vi "add control module.vi"(6 "output range":cluster{"output high":dbl, "output low":dbl}={"output high"=100.0, "output low"=-100.0}, 8 "error in":errorcluster, 9 "gains":T2, 10 "name":string, 11 "user module configuration in":refnum<class "TEST CONFIGURATION.lvclass">) -> (0 "error out":errorcluster, 1 "generated control module":T1={"name"="", "setpoint"=refnum, "process variable"=refnum, "output"=refnum, "gains"={"Kp"=0.0, "Ki"=0.0, "Kd"=0.0}, "output range"={"output high"=100.0, "output low"=-100.0}} {"output range"."output low" format="%.2f"; "output range"."output high" format="%.2f"}, 2 "generated channels":refnum<class "TBM channel.lvclass">[](array[class]), 3 "user module configuration out":refnum<class "TEST CONFIGURATION.lvclass">)   [LabVIEW 2013, in "configuration tests.lvlib" / "TEST CONFIGURATION.lvclass"]
uses:
  TEST CONFIGURATION.lvclass
  <vilib>/NI/Tag Bus Module Framework/channel/TBM channel.lvclass
  gains.ctl
  control module configuration.ctl
  TEST CONFIGURATION.lvclass/TEST CONFIGURATION.ctl
  <vilib>/NI/Tag Bus Module Framework/channel/channel classification.ctl
  <vilib>/NI/Tag Bus/tag/Data Type.ctl
  <vilib>/NI/Tag Bus/tag/tag descriptor.lvclass
  <vilib>/NI/Configuration Framework/NISE_CEF_TreeControl.lvlib
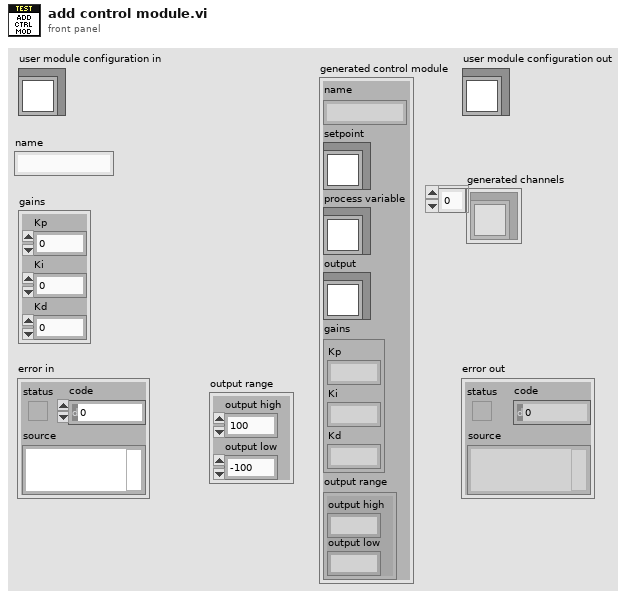
[diagram p1: front panel]
types:
  T1 = typedef "configuration tests.lvlib/TEST CONFIGURATION.lvclass/control module configuration.ctl" = cluster{"name":string, "setpoint":refnum<class "TBM channel.lvclass">, "process variable":refnum<class "TBM channel.lvclass">, "output":refnum<class "TBM channel.lvclass">, "gains":T2, "output range":cluster{"output high":dbl, "output low":dbl}}
  T2 = typedef "configuration tests.lvlib/TEST CONFIGURATION.lvclass/gains.ctl" = cluster{"Kp":dbl, "Ki":dbl, "Kd":dbl}
  T3 = typedef "TBM channel.lvclass/channel classification.ctl" = enum16{"input data", "output data", "processing parameter", "processing result"}
  T4 = typedef "tag bus.lvlib/tag descriptor.lvclass/Data Type.ctl" = enum16{"Double", "Single", "I64", "I32", "I16", "I8", "U64", "U32", "U16", "U8", "Boolean", "String", "Array of Double", "Array of Single", "Array of I64", "Array of I32", "Array of I16", "Array of I8", "Array of U64", "Array of U32", "Array of U16", "Array of U8", "Array of Boolean", "Array of String"}
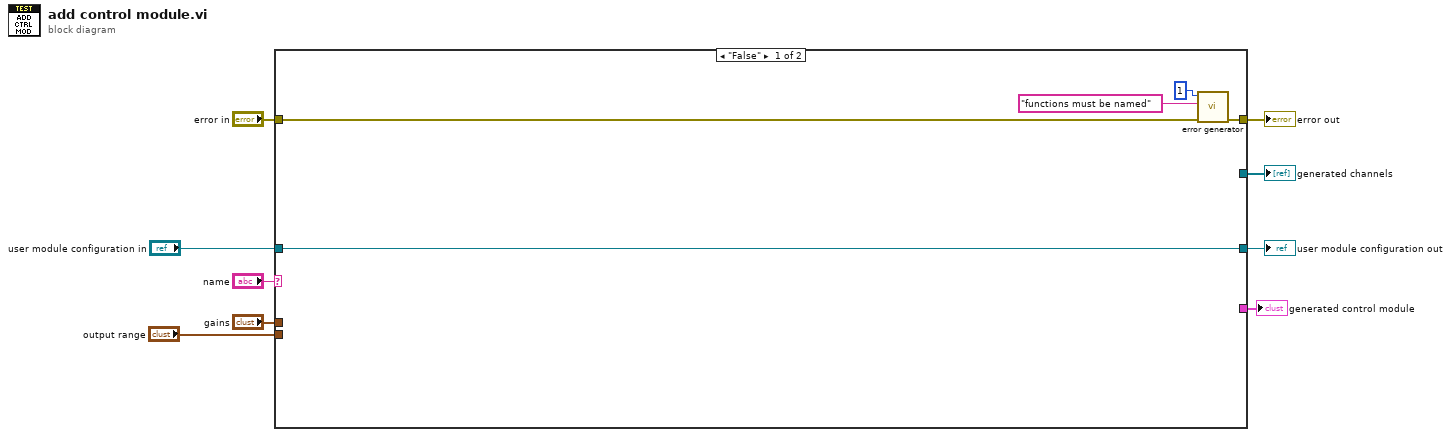
[diagram p0: block diagram]
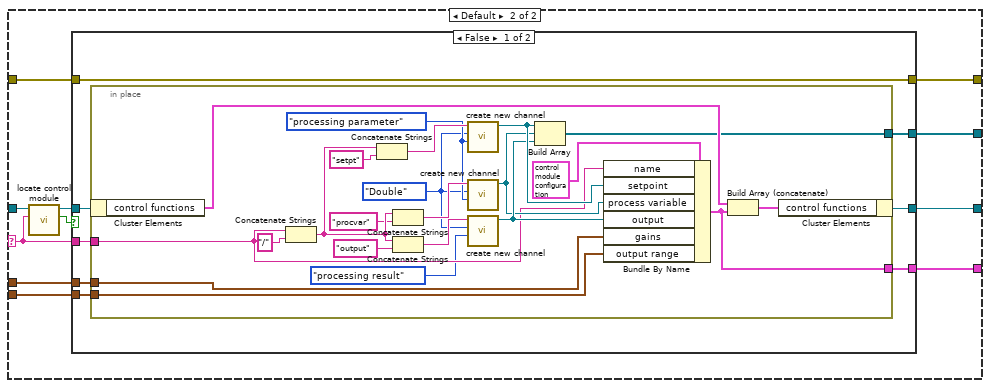
[diagram p2: hidden frame]
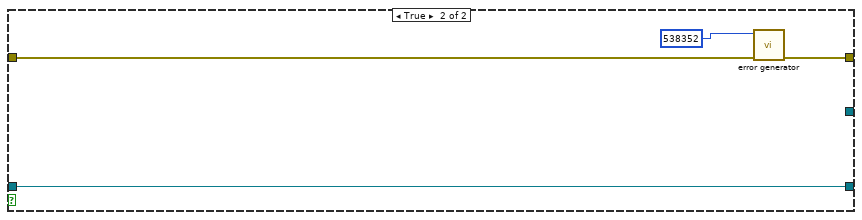
[diagram p3: hidden frame]
diagram:
  n1 = case shown="\"False\"" "name" {
    selector: "name" -> [_ w16]
    tunnel: "user module configuration in" -> [w14 w25]
    tunnel: "error in" -> [w13 w22]
    tunnel: [w12 w21] -> w7
    tunnel: [w14 w20] -> w6
    tunnel: [_ w19] -> w5
    tunnel: "output range" -> [_ w18]
    tunnel: "gains" -> [_ w17]
    tunnel: [_ w15] -> w1
    frame "False" {
      n2 = call <vilib>:"error generator.vi"("error in"=w13, "append error message"="functions must be named" ("error message (\"\")"), "error code (0)"=1) -> ("error out"=w12:errorcluster)  [unwired: 6 in]
    }
    frame Default {
      n3 = call "locate control module.vi"("name"=w16, "user module configuration in"=w25) -> ("found"=w23:bool, "user module configuration out"=w24:refnum<class "TEST CONFIGURATION.lvclass">)  [unwired: 6 in, 2 out]
      n4 = case shown="False" w23 {
        tunnel: w24 -> [w33 w56]
        tunnel: w22 -> [w31 w59]
        tunnel: [w31 w57] -> w21
        tunnel: [w32 w56] -> w20
        tunnel: w16 -> [w30 _]
        tunnel: [w29 _] -> w19
        tunnel: w18 -> [w28 _]
        tunnel: w17 -> [w27 _]
        tunnel: [w26 _] -> w15
        frame False {
          n5 = in-place {
            in-place-border: w30 -> [w48]
            in-place-border: [w49] -> w29
            in-place-border: w28 -> [w36]
            in-place-border: w27 -> [w35]
            in-place-border: [w34] -> w26
            w38 = Data_Type."Double" ("data type")
            w39 = channel_classification."processing parameter" ("channel classification")
            n6 = in-place-cluster #1(w33) -> ("control functions"=w54:T1[])
            n7 = Concatenate Strings(w48, "/" ("string")) -> (w46:string)
            n8 = Concatenate Strings(w46, "setpt" ("string")) -> (w40:string)
            n9 = Concatenate Strings(w46, "procvar" ("string")) -> (w41:string)
            n10 = Concatenate Strings(w46, "output" ("string")) -> (w42:string)
            n11 = call <vilib>:"create new channel.vi"("channel classification"=w39, "data type"=w38, "channel name"=w40) -> ("channel"=w52:refnum<class "TBM channel.lvclass">)  [unwired: 8 in]
            n12 = call <vilib>:"create new channel.vi"("channel classification"=w39, "data type"=w38, "channel name"=w41) -> ("channel"=w50:refnum<class "TBM channel.lvclass">)  [unwired: 8 in]
            n13 = call <vilib>:"create new channel.vi"("channel classification"=channel_classification."processing result", "data type"=w38, "channel name"=w42) -> ("channel"=w51:refnum<class "TBM channel.lvclass">)  [unwired: 8 in]
            n14 = Build Array(w52, w50, w51) -> (w49:refnum<class "TBM channel.lvclass">[])
            n15 = Bundle By Name(cluster=T1 {"name"="", "setpoint"=refnum, "process variable"=refnum, "output"=refnum, "gains"={"Kp"=0.0, "Ki"=0.0, "Kd"=0.0}, "output range"={"output high"=0.0, "output low"=0.0}} ("control module configuration"), "name"=w48, "setpoint"=w52, "process variable"=w50, "output"=w51, "gains"=w35, "output range"=w36) -> (w34:T1)
            n16 = Build Array (concatenate)(w54, w34) -> (w55:T1[])
            n17 = in-place-cluster #1("control functions"=w55) -> (w32:refnum<class "TEST CONFIGURATION.lvclass">)
          }
        }
        frame True {
          n18 = call <vilib>:"error generator.vi"("error in"=w59, "error code (0)"=538352) -> ("error out"=w57:errorcluster)  [unwired: 7 in]
        }
      }
    }
  }
  "error out" <- w7
  "user module configuration out" <- w6
  "generated channels" <- w5
  "generated control module" <- w1
